vi "Position Rest of Row.vi"(8 "Error In":errorcluster, 10 "First key in Row":refnum<vi>, 11 "Key Refs":refnum<vi>[](array[refnum])) -> (0 "Error Out":errorcluster)   [LabVIEW 2014]
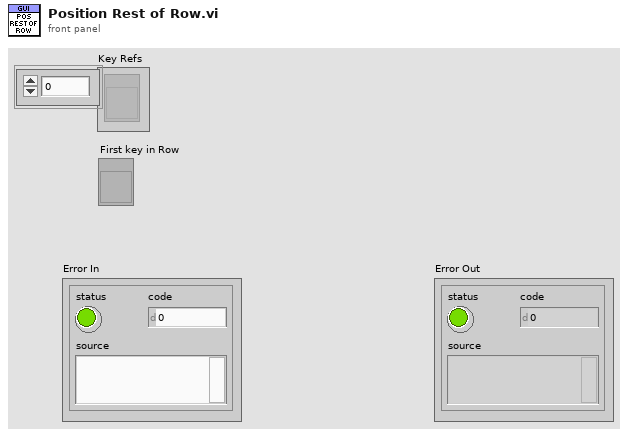
[diagram p1: front panel]
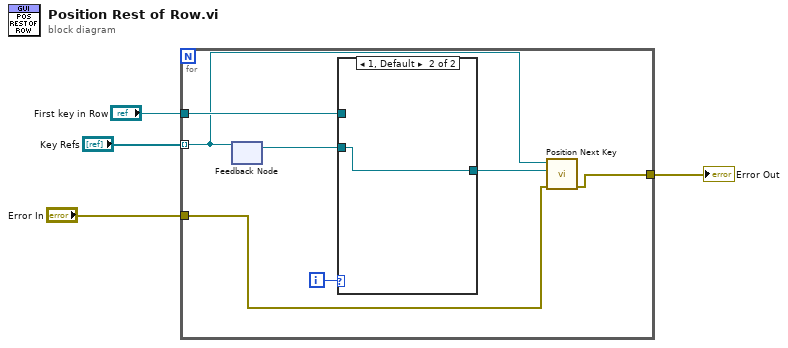
[diagram p0: block diagram]
diagram:
  n1 = for {
    tunnel: "Key Refs" -> [w6] mode=indexing
    tunnel: "Error In" -> [w8]
    tunnel: "First key in Row" -> [w10]
    tunnel: [w5] -> w1
    i -> [w11]
    n2 = feedback-in #1(w6) -> ()
    n3 = feedback #1() -> (w9:refnum<vi>)  [unwired: 1 in]
    n4 = case shown="1, Default" w11 {
      tunnel: w10 -> [w12 _]
      tunnel: w9 -> [_ w13]
      tunnel: [w12 w13] -> w7
      frame 0 {
        # "Use first key"
      }
      frame 1, Default {
      }
    }
    n5 = call "Position Next Key.vi"("error in (no error)"=w8, "Previous Key"=w7, "Input Key"=w6) -> ("error out"=w5:errorcluster)  [unwired: 8 in]
  }
  "Error Out" <- w1
